vi "Actor Core.vi"(8 "error in":errorcluster, 11 "Help in":refnum<class "Help.lvclass">) -> (0 "error out":errorcluster, 3 "Actor out":refnum<class "Actor.lvclass">)   [LabVIEW 2023, in "GUI.lvlib" / "Help.lvlib" / "Help.lvclass"]
doc: "(<B>Filename</B>: Actor Framework.lvlib:Actor.lvclass:Actor Core.vi)\n\nReceives messages to the actor, reacts to them, and initiates any error handling that may shut the actor down.\n\nDescendant classes may override this VI to append parallel tasks for the actor to complete while it handles messages. Overrides use the Call Parent Method node."
uses:
  Help.lvclass
  <vilib>/ActorFramework/Actor/Actor.lvclass
  <vilib>/ActorFramework/Actor/Actor.lvclass/Actor.ctl
  <vilib>/ActorFramework/Message Enqueuer/Message Enqueuer.lvclass/Message Enqueuer.ctl
  Reused Code/Subpanels Actor/subpanels/subpanel Messages/Insert Msg/Insert Msg.lvclass/Insert Msg.ctl
  <vilib>/ActorFramework/Message Enqueuer/Init from Existing Queue.vi
  <vilib>/ActorFramework/Message Enqueuer/Enqueue.vi
  Reused Code/Subpanels Actor/subpanels/subpanel Messages/Insert Msg/Insert Msg.lvclass
  <vilib>/ActorFramework/Message Priority Queue/Priority Enqueue.vi
  <vilib>/ActorFramework/Message Enqueuer/Message Enqueuer.lvclass
  Reused Code/Subpanels Actor/subpanels/subpanel/subpanel (abstract).lvclass
  HardwareAbstractionLayer_LVOOP/Error Handler/Error Handler_class/Error Handler.lvclass
panel:
  out "Boolean 2":bool
  in  "Boolean":bool
  in  "Stop":bool
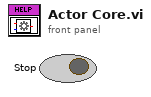
[diagram p1: front panel]
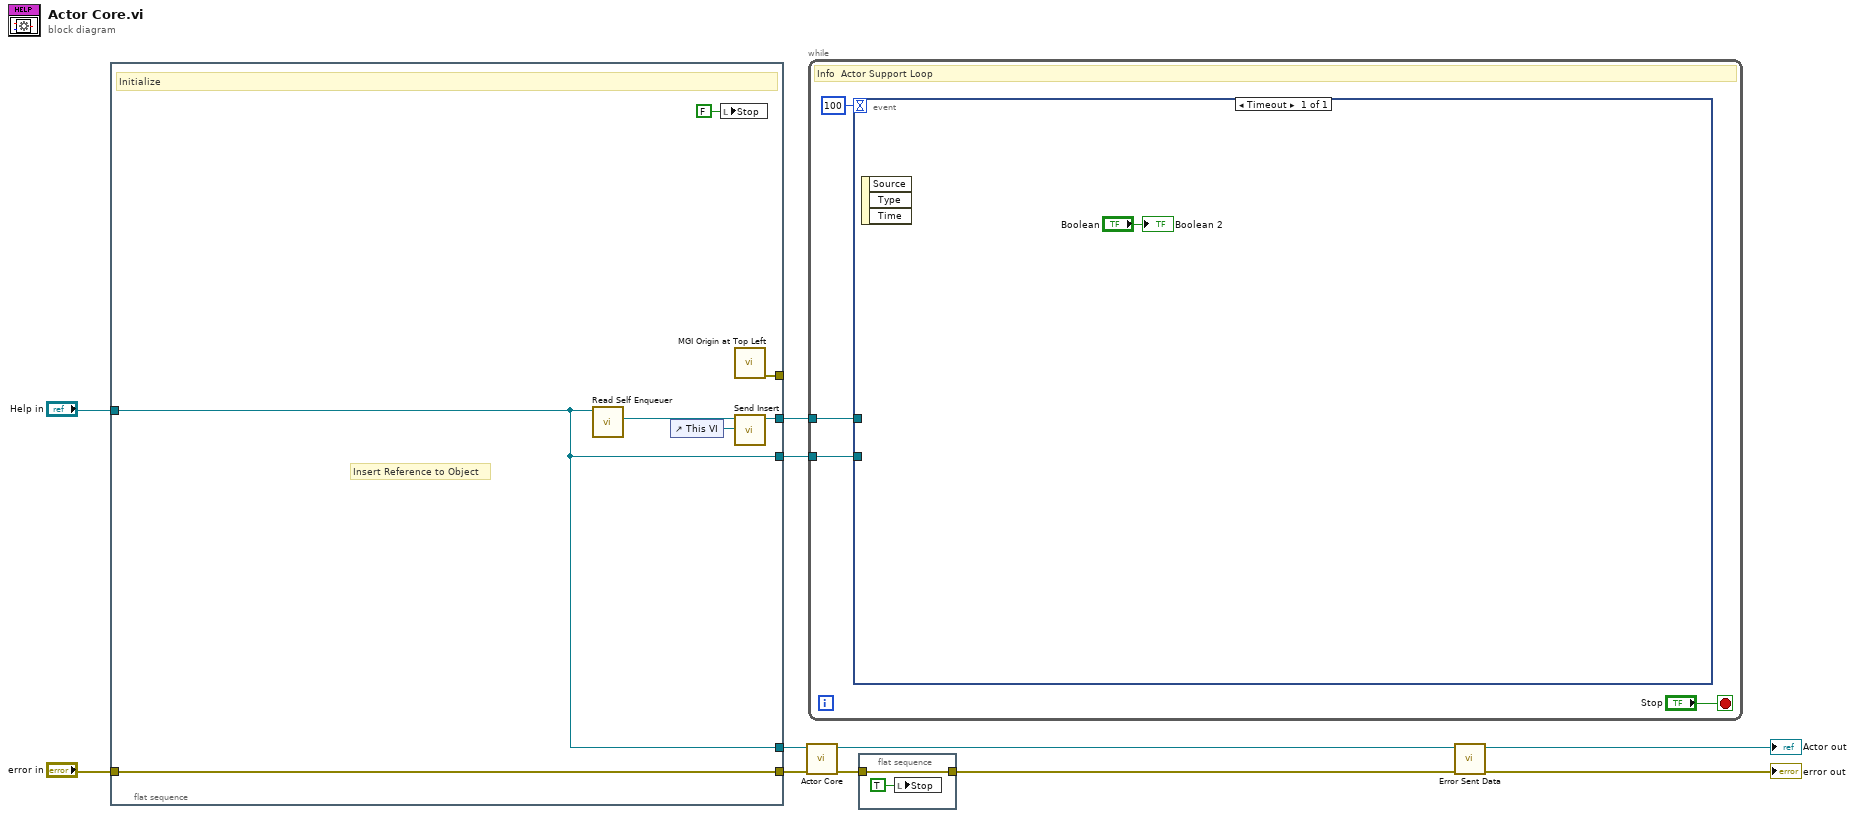
[diagram p0: block diagram]
diagram:
  n1 = flat-sequence {
    tunnel: "Help in" -> [w15]
    tunnel: [w13] -> w9
    tunnel: [w15] -> w8
    tunnel: [w17] -> w7
    tunnel: "error in" -> [w17]
    tunnel: [w16] -> _
    tunnel: [w15] -> w6
    frame #0 {
      # "Insert Reference to Object"
      # "Initialize"
      n2 = call <vilib>:"Read Self Enqueuer.vi"("Actor"=w15) -> ("Self Enqueuer"=w14:refnum<class "Message Enqueuer.lvclass">)  [unwired: 10 in]
      n3 = control-ref of="This VI"() -> (w12:refnum<vi>)
      n4 = local write "Stop"(FALSE ("Stop")) -> ()
      n5 = call <userlib>:"MGI Origin at Top Left.vi"() -> ("Error Out"=w16:errorcluster)  [unwired: 9 in, 1 out]
      n6 = call "Send Insert.vi"("VI Ref"=w12, "Message Enqueuer"=w14) -> ("Message Enqueuer out"=w13:refnum<class "Message Enqueuer.lvclass">)  [unwired: 8 in, 1 out]
    }
  }
  n7 = call-parent "Actor Core.vi"("error in"=w7, "Actor in"=w8) -> ("error out"=w10:errorcluster, "Actor out"=→"Actor out":refnum<class "Actor.lvclass">)  [unwired: 8 in]
  n8 = while {
    tunnel: w9 -> [w19]
    tunnel: w6 -> [w18]
    stop <- "Stop" stop-if-true
    # "Info  Actor Support Loop"
    n9 = event shown="[0] Timeout" {
      selector: _ -> [_]
      dyn-events: _ -> [_]
      timeout: 100 -> [_]
      tunnel: w19 -> [_]
      tunnel: w18 -> [_]
      event Timeout {
        n10 = event-data() -> ()  [unwired: 1 in, 3 out]
        "Boolean 2" <- "Boolean"
      }
    }
  }
  n11 = flat-sequence {
    tunnel: w10 -> [w24]
    tunnel: [w24] -> w2
    frame #0 {
      n12 = local write "Stop"(TRUE ("Stop")) -> ()
    }
  }
  n13 = call "Error Sent Data.vi"("error in"=w2) -> ("error out"=→"error out":errorcluster)  [unwired: 10 in]
